vi "save_to_db.vi"(3 "error in":errorcluster, 5 "Raw Signal 3":waveform(dbl)[](array[waveform])) -> (0 "error out":errorcluster)   [LabVIEW 2018]
uses:
  <vilib>/drjdpowell/SQLite Library/SQL Statement/SQL Statement.lvclass/SQL Statement.ctl
  <vilib>/drjdpowell/SQLite Library/SQL Connection/Open (path).vi
  <vilib>/drjdpowell/SQLite Library/SQL Statement/Bind Real.vi
  <vilib>/drjdpowell/SQLite Library/SQL Connection/Open (string).vi
  <vilib>/drjdpowell/SQLite Library/SQL Statement/Step.vi
  <vilib>/AdvancedString/Path To Command Line String.vi
  <vilib>/drjdpowell/SQLite Library/SQL Statement/Error Message.vi
  <vilib>/drjdpowell/SQLite Library/SQL Connection/Connection.lvclass
  <vilib>/drjdpowell/SQLite Library/SQL Statement/SQL Statement.lvclass
  <vilib>/drjdpowell/SQLite Library/Transaction Helpers/Transaction.lvlib
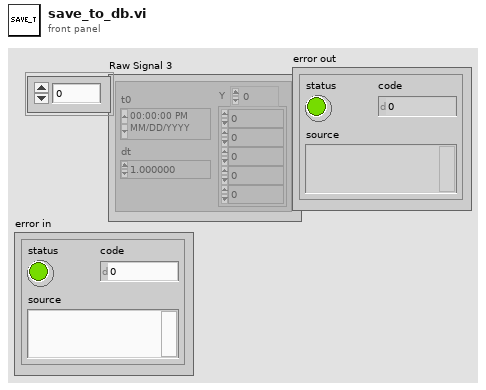
[diagram p1: front panel]
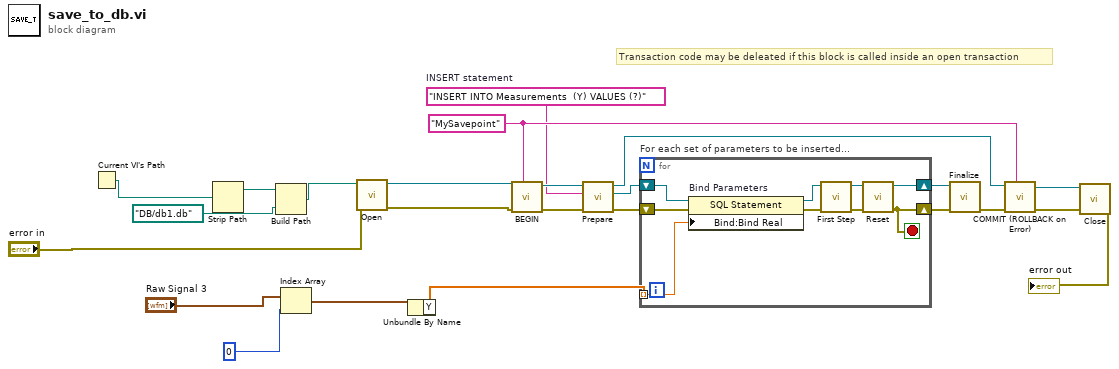
[diagram p0: block diagram]
diagram:
  w18 = "MySavepoint" ("Savepoint name")
  w13 = "INSERT INTO Measurements  (Y) VALUES (?)"  # INSERT statement
  # "Transaction code may be deleated if this block is called inside an open transaction"
  n1 = Current VI's Path() -> (path=w24:path)
  n2 = Strip Path(path=w24) -> (stripped path=w23:path)  [unwired: 1 out]
  n3 = Build Path(base path=w23, name or relative path=path "DB/db1.db") -> (appended path=w22:path)
  n4 = Index Array(array="Raw Signal 3", index=0) -> (element=w6:waveform(dbl))
  n5 = call-poly <vilib>:"Open.vi"("error in (no error)"="error in", "db file"=w22) -> ("error out"=w3:errorcluster, "SQLite Connection"=w10:refnum<class "Connection.lvclass">)  [unwired: 8 in]
  n6 = Unbundle By Name(w6) -> ("Y"=w5:dbl[])
  n7 = call <vilib>:"BEGIN.vi"("Savepoint name"=w18, "error in (no error)"=w3, "SQLite Connection in"=w10) -> ("error out"=w17:errorcluster, "SQLite Connection"=w16:refnum<class "Connection.lvclass">)  [unwired: 7 in]
  n8 = call <vilib>:"Prepare.vi"("error in (no error)"=w17, "SQL"=w13, "SQLite Connection in"=w16) -> ("error out"=w12:errorcluster, "SQL Statement"=w11:refnum<class "SQL Statement.lvclass">, "SQLite Connection"=w19:refnum<class "Connection.lvclass">)  [unwired: 4 in, 2 out]
  n9 = for "For each set of parameters to be inserted..." {
    shift-right: [w27] -> w14
    shift-left: w11 -> [w33]
    shift-right: [w26] -> w15
    shift-left: w12 -> [w30]
    tunnel: w5 -> [w25] mode=indexing
    stop <- w26 stop-if-true
    n10 = property on="Bind Parameters" class="SQL Statement"(reference=w33, error in=w30, "Bind:Bind Real"=w25) -> (reference out=w32:refnum<class "SQL Statement.lvclass">, error out=w31:errorcluster)
    n11 = call <vilib>:"First Step.vi"("error in (no error)"=w31, "SQL Statement in"=w32) -> ("error out"=w29:errorcluster, "SQL Statement"=w28:refnum<class "SQL Statement.lvclass">)  [unwired: 7 in, 1 out]
    n12 = call <vilib>:"Reset.vi"("error in (no error)"=w29, "SQL Statement in"=w28) -> ("error out"=w26:errorcluster, "SQL Statement"=w27:refnum<class "SQL Statement.lvclass">)  [unwired: 8 in]
  }
  n13 = call <vilib>:"Finalize.vi"("error in (no error)"=w15, "SQL Statement in"=w14) -> ("error out"=w20:errorcluster)  [unwired: 9 in]
  n14 = call <vilib>:"COMMIT (ROLLBACK on Error).vi"("Savepoint name"=w18, "error in (no error)"=w20, "SQLite Connection in"=w19) -> ("error out"=w2:errorcluster, "SQLite Connection"=w9:refnum<class "Connection.lvclass">)  [unwired: 7 in]
  n15 = call-dynamic "Close.vi"("error in (no error)"=w2, "SQLite Connection in"=w9) -> ("error out"=→"error out":errorcluster)  [unwired: 9 in]
